vi "Contador 0-9.vi"() -> ()   [LabVIEW 2022 SP3]
panel:
  in  "Up":bool
  in  "s/p":bool
  out "Numeric":u32
  in  "T":bool
  in  "Start/Pause":bool
  in  "Reset":bool
  in  "Stop":bool
  out "e":bool
  out "f":bool
  out "c":bool
  out "b":bool
  out "d":bool
  out "g":bool
  out "a":bool
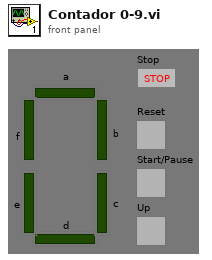
[diagram p1: front panel]
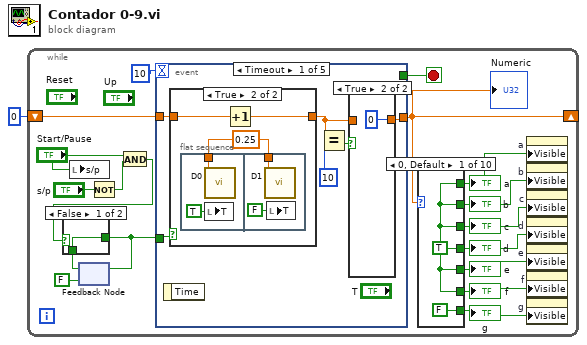
[diagram p0: block diagram]
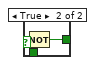
[diagram p2: hidden frame]
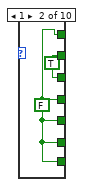
[diagram p3: hidden frame]
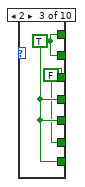
[diagram p4: hidden frame]
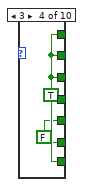
[diagram p5: hidden frame]
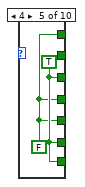
[diagram p6: hidden frame]
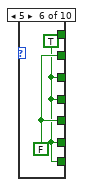
[diagram p7: hidden frame]
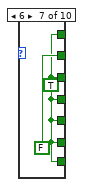
[diagram p8: hidden frame]
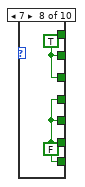
[diagram p9: hidden frame]
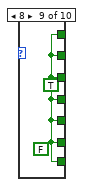
[diagram p10: hidden frame]
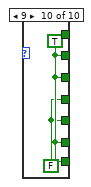
[diagram p11: hidden frame]
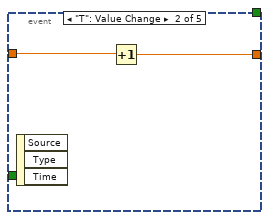
[diagram p14: hidden frame]
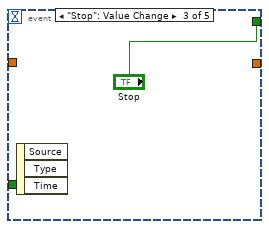
[diagram p15: hidden frame]
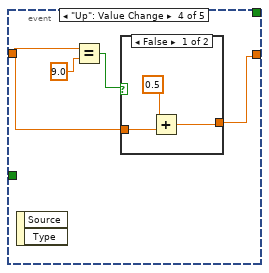
[diagram p16: hidden frame]
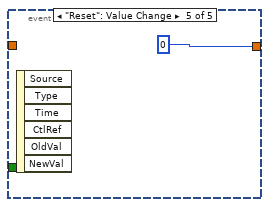
[diagram p18: hidden frame]
diagram:
  n1 = while {
    shift-right: [w2] -> _
    shift-left: u16 0 -> [w19]
    stop <- w18 stop-if-true
    n2 = local write "s/p"("Start/Pause") -> ()
    n3 = feedback #1(FALSE) -> (w4:bool)
    n4 = Not(x="s/p") -> (.not. x?=w7:bool)
    n5 = And(x="Start/Pause", y=w7) -> (x .and. y?=w6:bool)
    n6 = case shown="False" w6 {
      tunnel: [w20 w22] -> w5
      tunnel: w4 -> [w20 w21]
      frame False {
      }
      frame True {
        n7 = Not(x=w21) -> (.not. x?=w22:bool)
      }
    }
    n8 = feedback-in #1(w5) -> ()
    n9 = event shown="[0] Timeout" {
      selector: _ -> [_ _ _ _ _]
      dyn-events: _ -> [_ _ _ _ _]
      timeout: 10 -> [_ _ _ _ _]
      tunnel: w19 -> [w47 w58 _ w61 _]
      tunnel: [w44 w59 _ w62 0] -> w2
      tunnel: [_ _ "Stop" _ _] -> w18
      tunnel: w5 -> [w42 _ _ _ _]
      event Timeout {
        n10 = event-data() -> ()  [unwired: 1 in, 1 out]
        n11 = case shown="True" w42 {
          tunnel: w47 -> [w50 w52]
          tunnel: [w50 w51] -> w43
          frame False {
          }
          frame True {
            w53 = 0.25
            n12 = flat-sequence {
              tunnel: w53 -> [w54]
              tunnel: w53 -> [w56]
              frame #0 {
                n13 = call "D0"("Delay Time (s)"=w54) -> ()  [unwired: 10 in, 1 out]
                n14 = local write "T"(TRUE) -> ()
              }
              frame #1 {
                n15 = call "D1"("Delay Time (s)"=w56) -> ()  [unwired: 10 in, 1 out]
                n16 = local write "T"(FALSE) -> ()
              }
            }
            n17 = Increment(x=w52) -> (x+1=w51:dbl)
          }
        }
        n18 = Equal?(x=w43, y=10) -> (x = y?=w46:bool)
        n19 = case shown="True" w46 {
          tunnel: [w48 0] -> w44
          tunnel: w43 -> [w48 _]
          frame False {
          }
          frame True {
          }
        }
      }
      event "T": Value Change {
        n20 = event-data() -> ()  [unwired: 1 in, 3 out]
        n21 = Increment(x=w58) -> (x+1=w59:dbl)
      }
      event "Stop": Value Change {
        n22 = event-data() -> ()  [unwired: 1 in, 3 out]
      }
      event "Up": Value Change {
        n23 = event-data() -> ()  [unwired: 1 in, 2 out]
        n24 = Equal?(x=w61, y=9.0) -> (x = y?=w63:bool)
        n25 = case shown="False" w63 {
          tunnel: [w67 w68] -> w62
          tunnel: w61 -> [w65 w68]
          frame False {
            n26 = Add(x=0.5, y=w65) -> (x+y=w67:dbl)
          }
          frame True {
          }
        }
      }
      event "Reset": Value Change {
        n27 = event-data() -> ()  [unwired: 1 in, 6 out]
      }
    }
    "Numeric" <- w2
    n28 = case shown="0, Default" w2 {
      tunnel: [w24 w25 w28 w30 w31 w33 w35 w38 w39 w41] -> w15
      tunnel: [w24 w26 w28 w30 w32 w34 FALSE w38 w39 w41] -> w16
      tunnel: [w24 w26 w27 w30 w32 w33 w35 w38 w39 w41] -> w14
      tunnel: [w24 w25 w28 w30 w31 w33 w35 w37 w39 w40] -> w13
      tunnel: [w24 w25 w28 w29 w31 w34 w35 w37 w39 w40] -> w12
      tunnel: [w24 w25 w27 w29 w32 w33 w35 w37 w39 w41] -> w11
      tunnel: [FALSE w25 w28 w30 w32 w33 w35 w37 w39 w41] -> w10
      frame 0, Default {
        w24 = TRUE
      }
      frame 1 {
        w25 = FALSE
        w26 = TRUE
      }
      frame 2 {
        w27 = FALSE
        w28 = TRUE
      }
      frame 3 {
        w29 = FALSE
        w30 = TRUE
      }
      frame 4 {
        w31 = FALSE
        w32 = TRUE
      }
      frame 5 {
        w34 = FALSE
        w33 = TRUE
      }
      frame 6 {
        w35 = TRUE
      }
      frame 7 {
        w37 = FALSE
        w38 = TRUE
      }
      frame 8 {
        (unwired) FALSE
        w39 = TRUE
      }
      frame 9 {
        w40 = FALSE
        w41 = TRUE
      }
    }
    "a" <- w15
    "g" <- w10
    "d" <- w13
    "b" <- w16
    "c" <- w14
    "f" <- w11
    "e" <- w12
    n29 = property on="a" class="Bool (strict)"("Visible"=w15) -> ()  [unwired: 2 in, 2 out]
    n30 = property on="b" class="Bool (strict)"("Visible"=w16) -> ()  [unwired: 2 in, 2 out]
    n31 = property on="c" class="Bool (strict)"("Visible"=w14) -> ()  [unwired: 2 in, 2 out]
    n32 = property on="d" class="Bool (strict)"("Visible"=w13) -> ()  [unwired: 2 in, 2 out]
    n33 = property on="e" class="Bool (strict)"("Visible"=w12) -> ()  [unwired: 2 in, 2 out]
    n34 = property on="f" class="Bool (strict)"("Visible"=w11) -> ()  [unwired: 2 in, 2 out]
    n35 = property on="g" class="Bool (strict)"("Visible"=w10) -> ()  [unwired: 2 in, 2 out]
  }
